vi "適應性控制_輸入權重係數+數位積分_隔振(實際控制).vi"() -> ()   [LabVIEW 2010]
uses:
  <vilib>/DAQmx/read.llb/DAQmx Read (Analog DBL 1Chan 1Samp).vi
  <vilib>/DAQmx/write.llb/DAQmx Write (Analog DBL 1Chan 1Samp).vi
  <vilib>/DAQmx/create/channels.llb/DAQmx Create Channel (AI-Voltage-Basic).vi
  <vilib>/DAQmx/configure/timing.llb/DAQmx Timing (Sample Clock).vi
  <vilib>/DAQmx/create/channels.llb/DAQmx Create Channel (AO-Voltage-Basic).vi
  <vilib>/daqmx/miscellaneous.llb/DAQmx Fill In Error Info.vi
  <vilib>/measure/maspectr.llb/FFT Spectrum (Mag-Phase) for 1 Chan.vi
  <vilib>/measure/NI_MAPro.lvlib
panel:
  in  "averaging parameters":T1={"averaging mode"=enum."No averaging", "weighting mode"=enum."Exponential", "number of averages"=10} {"number of averages" min=1}
  in  "I增益":dbl
  out "magnitude":cluster{"f0":dbl, "df":dbl, "magnitude":dbl[]} {"magnitude" format="%.2p"; "f0" format="%0.2p"; "df" format="%0.2p"}
  out "x >= y?":bool
  out "Waveform Graph":cluster{"f0":dbl, "df":dbl, "magnitude":dbl[]}(graph)
  in  "DAQ input":tag
  in  "DAQ output":tag
  in  "平均數":i32=1
  in  "ÂoDC«á©ñ¤j":dbl=1.0
  in  "Kp":dbl
  out "當下誤差":dbl=0.1 format="%#_13g"
  out "模擬輸入x(t)":dbl[][](graph)
  out "理想與FIR輸出":dbl[][](graph)
  out "message":string=" INSTRUCTIONS:\r\rNormal Use:  When using subVIs that incorporate the error in/error out (or error I/O) structure, place this handler where you want to inform the user of an error, typically at the end of the I/O data path, as the last action of the program.  If the error in error? is ERROR, the handler creates a message describing the error and its source.  If the type of dialog = 1 (default), the message is displayed to the user, who can only acknowedge it.  If the type = 2, the user can acknowledge the message or abort execution; aborting a program with active I/O is not recommended.  If the type = 0, no message is displayed; this is used to process the error programmatically, and the error out cluster elements are wired to individual terminals for that reason.  \r\rOther Use:\n\r\nlocal testing.  To test the error code of a subVI or function that does not have the error I/O structure, you can wire its error code and a source string to the local error code and error source inputs.  If error in error? indicates no error and error code is not equal to 0, the local code and source are substituted for the error in values, and error? is set TRUE (ERROR)."
  out "誤差":dbl(graph)
  out "while平均運行時間":dbl
  out "收斂time":dbl
  out "各頻率誤差已達標準":bool
  in  "各頻率誤差低於多少亮燈":dbl=0.1 format="%#_13g"
  in  "order":i32=100
  in  "取樣頻率":dbl=100.0 min=1.0 max=1000.0 step=1.0
  in  "stop":bool
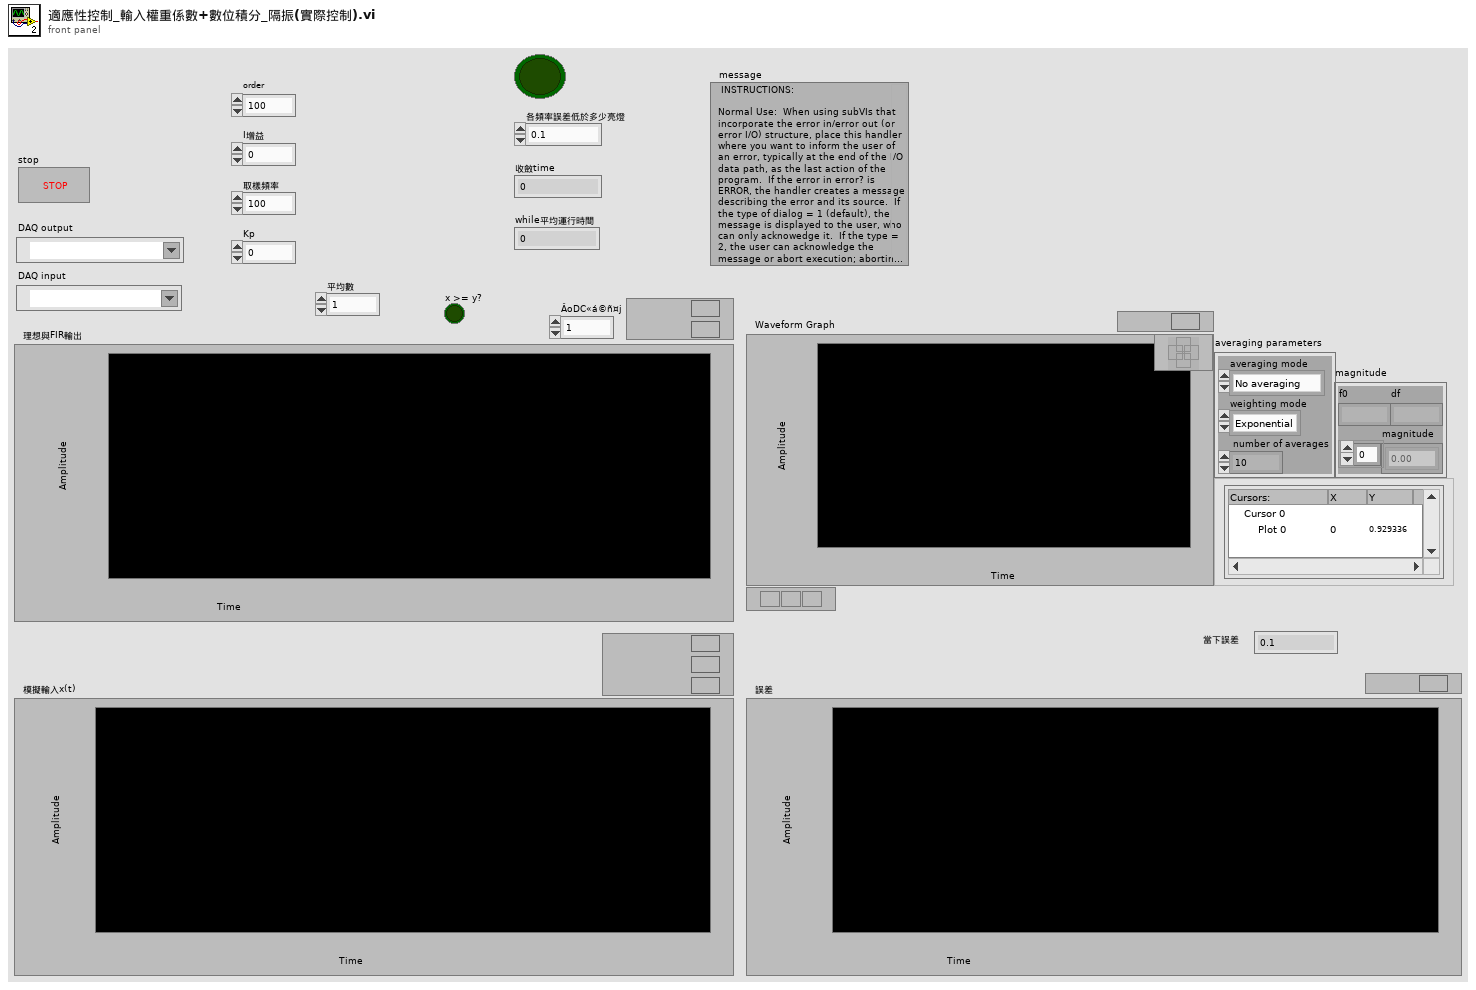
[diagram p1: front panel]
types:
  T1 = cluster{"averaging mode":enum16{"No averaging", "Vector averaging", "RMS averaging", "Peak hold"}, "weighting mode":enum16{"Linear", "Exponential"}, "number of averages":u32}
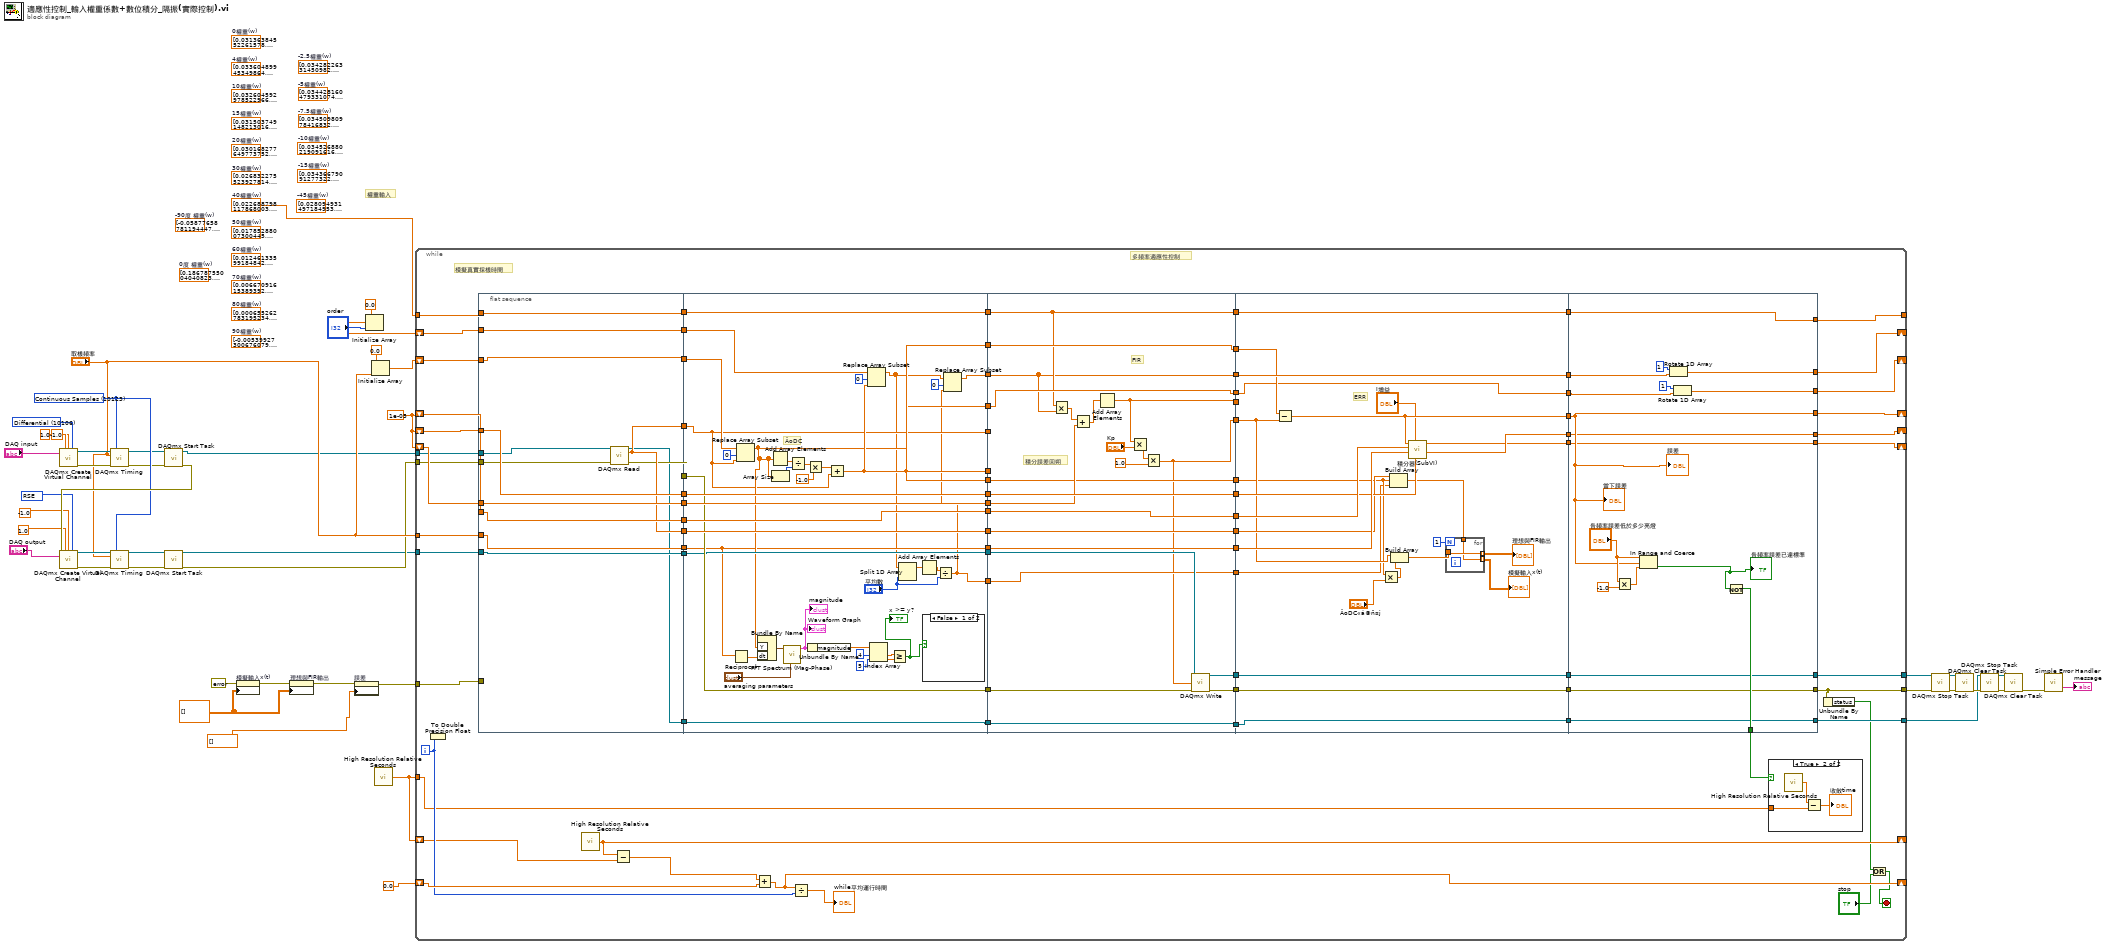
[diagram p0: block diagram]
diagram:
  (unwired) dbl[] [0.028094931497184953, 0.027318051498735518, 0.02651879137319172, 0.02569807185586792, 0.024856829443012252, 0.023996015437237974, 0.023116594986324603, 0.022219546115147443, 0.021305858750507205, 0.020376533738653148, 0.019432581855336542, 0.01847502280827197, 0.01750488423195552, 0.01652320067484008, 0.015531012578964592, 0.014529365252202192, 0.013519307833396409, 0.012501892250745314, 0.011478172173896465, 0.010449201960325366, 0.009416035596672211, 0.00837972563582886, 0.007341322130674419, 0.0063018715654710395, 0.005262415786041815, 0.004223990929959873, 0.003187626358084177, 0.002154343588880318, 0.0011251552370595153, 0.00010106395816484767, -0.0009169385991820944, -0.001927872831580498, -0.002930772207829844, -0.00392468428265997, -0.004908671695227361, -0.00588181315034755, -0.006843204380400101, -0.007791959085817819, -0.008727209852058984, -0.009648109040964999, -0.010553829654414855, -0.011443566168217257, -0.012316535334218085, -0.013171976948660059, -0.014009154584890944, -0.014827356288608607, -0.015625895233920068, -0.016404110338605567, -0.017161366837102645, -0.017897056809864115, -0.018610599667884493, -0.019301442591371253, -0.019969060921687886, -0.020612958505892797, -0.021232667993384594, -0.02182775108436404, -0.022397798730027247, -0.02294243128460723, -0.02346129860960119, -0.023954080130721905, -0.024420484848320073, -0.02486025130223469, -0.025273147492222828, -0.025658970755303042, -0.026017547601540937, -0.026348733509958266, -0.026652412686409777, -0.02692849778540182, -0.02717692959795794, -0.02739767670772351, -0.027590735117597045, -0.027756127849228453, -0.027893904517764606, -0.02800414088424619, -0.028086938388049064, -0.028142423661741165, -0.028170748030678785, -0.02817208699960081, -0.028146639728389652, -0.02809462849906762]  # -45權重(w)
  (unwired) dbl[] [-0.00539927300676079, -0.004574244171263112, -0.0037509801609765317, -0.0029302816336518054, -0.002112938043582804, -0.0012997269243527085, -0.0004914132117880658, 0.00031125139289816275, 0.001107529020049304, 0.00189669618911319, 0.0026780443275469003, 0.003450880252045411, 0.004214526613258243, 0.004968322305336847, 0.005711622841811576, 0.006443800699430544, 0.007164245631703628, 0.00787236495397947, 0.008567583801947519, 0.009249345365491084, 0.00991711109983541, 0.01057036091592068, 0.01120859335190286, 0.011831325727629191, 0.01243809428386606, 0.013028454307965948, 0.013601980247555422, 0.014158265813706777, 0.014696924074924332, 0.015217587543133453, 0.015719908252715378, 0.01620355783346848, 0.016668227578224903, 0.017113628505685517, 0.01753949141887445, 0.01794556695946006, 0.01833162565802534, 0.018697457980225856, 0.019042874368621635, 0.01936770527983496, 0.019671801216557375, 0.019955032753801623, 0.02021729055869038, 0.02045848540297177, 0.020678548167360374, 0.02087742983672937, 0.021055101485111045, 0.02121155424941127, 0.021346799290705574, 0.02146086774194928, 0.02155381064092829, 0.02162569884726334, 0.021676622942297136, 0.02170669311070986, 0.02171603900274138, 0.02170480957594453, 0.021673172915446008, 0.021621316031757785, 0.02154944463526281, 0.0214577828865742, 0.021346573122078515, 0.021216075554065406, 0.02106656794496731, 0.02089834525535277, 0.0207117192654478, 0.020507018170093982, 0.02028458614719378, 0.020044782899845154, 0.019787983172514116, 0.019514576241749453, 0.019224965382103488, 0.01891956730807669, 0.018598811593062675, 0.01826314006642601, 0.017913006189998734, 0.017548874415424298, 0.017171219523929186, 0.01678052595022868, 0.016377287092401892, 0.015962004609691362]  # 90權重(w)
  (unwired) dbl[] [0.000655262783195234, 0.0014201078745085935, 0.0021774020972579466, 0.002926443888983223, 0.0036665482827068136, 0.004397047528653455, 0.005117291670540145, 0.005826649076006129, 0.006524506921026103, 0.0072102716284213626, 0.007883369260847498, 0.008543245868894885, 0.009189367795184315, 0.009821221935571046, 0.010438315958788755, 0.011040178486057891, 0.011626359232366039, 0.012196429111279456, 0.012749980305275018, 0.01328662630369608, 0.013806001910512301, 0.014307763224125022, 0.014791587591492175, 0.01525717353885328, 0.015704240681322403, 0.016132529613576106, 0.016541801783804003, 0.01693183935301074, 0.017302445041656855, 0.017653441965513737, 0.017984673462477143, 0.018296002911941722, 0.01858731354818533, 0.018858508269058803, 0.019109509441096958, 0.01934025870201465, 0.01955071676136483, 0.019740863199973476, 0.019910696268596727, 0.020060232686074937, 0.020189507437109056, 0.020298573569623023, 0.02038750199153626, 0.02045638126663941, 0.020505317409132445, 0.020534433676282337, 0.020543870358546826, 0.02053378456642888, 0.020504350013242287, 0.020455756792913834, 0.02038821115188715, 0.02030193525416185, 0.0201971669384727, 0.02007415946660244, 0.019933181261818818, 0.01977451563643863, 0.01959846050754766, 0.019405328099933034, 0.019195444635336765, 0.018969150007184216, 0.018726797440022064, 0.018468753132954787, 0.018195395886468565, 0.01790711671211353, 0.017604318424615885, 0.017287415216095867, 0.016956832212185698, 0.016613005009947363, 0.016256379197624637, 0.015887409856384125, 0.015506561044327013, 0.015114305263196064, 0.014711122908324714, 0.014297501702517113, 0.013873936114681207, 0.01344092676416721, 0.012998979811898303, 0.01254860633950505, 0.012090321717796058, 0.011624644966018761]  # 80權重(w)
  (unwired) dbl[] [0.00667091615389392, 0.0073531796215807205, 0.008022353499817968, 0.008677855658426154, 0.0093191252965615, 0.009945623446932242, 0.01055683343253673, 0.011152261275102226, 0.01173143605465801, 0.012293910219937266, 0.012839259849567968, 0.0133670848642776, 0.013877009190596819, 0.014368680876806187, 0.014841772162116167, 0.015295979500309196, 0.015731023539294408, 0.01614664905823473, 0.01654262486409535, 0.016918743649629534, 0.017274821814967204, 0.01761069925509673, 0.017926239115628573, 0.018221327519306194, 0.018495873265781063, 0.018749807507191584, 0.018983083402092395, 0.019195675750248362, 0.019387580610770918, 0.01955881490600148, 0.019709416013460674, 0.019839441348070867, 0.01994896793674781, 0.02003809198730413, 0.020106928453470334, 0.02015561059767175, 0.020184289553033544, 0.020193133885911513, 0.02018232916007052, 0.020152077503450435, 0.020102597178287, 0.02003412215517216, 0.019946901691477305, 0.019841199914387982, 0.019717295408651407, 0.019575480808984056, 0.0194160623969507, 0.019239359702002117, 0.019045705106238656, 0.01883544345237183, 0.018608931654259798, 0.018366538309320644, 0.01810864331206435, 0.017835637467933978, 0.017547922106607765, 0.0172459086938986, 0.016930018441365446, 0.016600681912763208, 0.0162583386264637, 0.015903436653009115, 0.015536432206992573, 0.01515778923250659, 0.014767978981454962, 0.014367479584085715, 0.013956775611178068, 0.013536357627390475, 0.013106721735366355, 0.012668369110286092, 0.012221805524647291, 0.011767540863162248, 0.011306088627763677, 0.010837965432821188, 0.01036369049078064, 0.009883785088553226, 0.009398772055093806, 0.008909175220725613, 0.00841551886887598, 0.007918327181006855, 0.007418123675629097, 0.006915430642395791]  # 70權重(w)
  (unwired) dbl[] [0.01246133599184842, 0.013041219831202504, 0.013602894406144423, 0.014145913686861338, 0.014669856948559828, 0.015174329133535792, 0.015658961166438435, 0.01612341022168393, 0.01656735994218592, 0.016990520608790343, 0.017392629260042803, 0.017773449762143567, 0.018132772829205633, 0.01847041599416169, 0.01878622353092701, 0.019080066328656997, 0.019351841719184283, 0.01960147325894746, 0.019828910466937345, 0.020034128520405686, 0.02021712791025534, 0.02037793405822041, 0.020516596898084622, 0.020633190423331605, 0.020727812203723175, 0.020800582873394126, 0.020851645593115937, 0.020881165489419887, 0.02088932907328999, 0.020876343641121745, 0.02084243666062208, 0.020787855144258918, 0.020712865012808217, 0.02061775045144026, 0.020502813260682387, 0.020368372204463133, 0.020214762357301148, 0.02004233445254702, 0.01985145423342024, 0.019642501808414096, 0.019415871012459316, 0.019171968775060666, 0.018911214496432904, 0.018634039432489067, 0.01834088608934769, 0.01803220762786084, 0.017708467278491697, 0.01737013776671445, 0.017017700748963114, 0.01665164625901359, 0.016272472164555577, 0.015880683633604304, 0.015476792610288682, 0.015061317299474863, 0.014634781659602443, 0.014197714903051736, 0.01375065100331456, 0.013294128208201897, 0.012828688558305545, 0.012354877409919147, 0.011873242961626859, 0.011384335783784626, 0.010888708350142303, 0.010386914570892993, 0.009879509326477619, 0.00936704800152902, 0.008850086018401487, 0.008329178369796334, 0.007804879150074156, 0.007277741084921289, 0.006748315059123063, 0.006217149642286703, 0.005684790612449048, 0.005151780477596648, 0.004618657995224534, 0.004085957690156384, 0.003554209370946196, 0.003023937645278717, 0.0024956614348826222, 0.0019698934905635845]  # 60權重(w)
  (unwired) dbl[] [0.01785288007300445, 0.018313549484099297, 0.01875146243947006, 0.019166321764041604, 0.01955785875766229, 0.019925833390966242, 0.020270034456919973, 0.02059027967701616, 0.02088641576122781, 0.021158318421011374, 0.021405892334826912, 0.021629071065836773, 0.021827816931648425, 0.02200212082617336, 0.02215200199389503, 0.0222775077570517, 0.022378713196462365, 0.022455720786945993, 0.022508659988498554, 0.02253768679459808, 0.022542983239220365, 0.022524756864332075, 0.022483240149813264, 0.02241868990792409, 0.022331386644584658, 0.022221633889865745, 0.022089757500200716, 0.021936104934927047, 0.021761044509828513, 0.021564964630406868, 0.021348273007631896, 0.021111395858927785, 0.020854777097133657, 0.020578877510134784, 0.02028417393380734, 0.019971158420829367, 0.01964033740782395, 0.01929223088316994, 0.018927371557704305, 0.01854630404037417, 0.018149584020758995, 0.017737777460210984, 0.017311459793187052, 0.016871215140176334, 0.016417635533441485, 0.015951320156614594, 0.01547287459900939, 0.014982910125334536, 0.014482042961323908, 0.013970893595633676, 0.013450086098201664, 0.012920247455119799, 0.012382006919929456, 0.011835995381132669, 0.011282844745594366, 0.010723187337414892, 0.010157655311766505, 0.00958688008311379, 0.009011491767180241, 0.008432118635978309, 0.007849386585186942, 0.007263918613140568, 0.006676334310689538, 0.006087249361190102, 0.0054972750499046215, 0.004907017782112015, 0.004317078609266263, 0.003728052762584605, 0.0031405291934967785, 0.0025550901204460315, 0.0019723105815968736, 0.0013927579930736271, 0.0008169917124283485, 0.0002455626071138371, -0.00032098737218195605, -0.0008821256134018418, -0.0014373292601635595, -0.0019860856238763302, -0.0025278925907399885, -0.0030622590233541505]  # 50權重(w)
  w1 = dbl[] [0.022688798117868003, 0.023016703123977605, 0.023318008487520508, 0.02359257453440416, 0.023840292415774466, 0.024061084118485853, 0.024254902434520387, 0.024421730888538103, 0.024561583622842255, 0.02467450523916157, 0.02476057059678428, 0.024819884566718728, 0.024852581741703586, 0.02485882610205748, 0.02483881063751958, 0.0247927569254129, 0.024720914665639287, 0.024623561173202368, 0.024501000829138836, 0.024353564490923844, 0.024181608863604643, 0.023985515833094145, 0.02376569176323148, 0.02352256675838937, 0.023256593893559507, 0.02296824841400089, 0.022658026906665633, 0.02232644644574225, 0.02197404371475412, 0.021601374107744833, 0.021209010812141927, 0.02079754387595296, 0.020367579261963257, 0.019919737891628254, 0.019454654681336437, 0.018972977573689306, 0.01847536656640235, 0.017962492741357045, 0.017435037296253165, 0.016893690581209736, 0.016339151142542342, 0.015772124775823664, 0.015193323590181596, 0.014603465085647513, 0.014003271245200621, 0.013393467642993524, 0.012774782570070415, 0.012147946178719771, 0.011513689646429045, 0.010872744360239406, 0.01022584112213084, 0.009573709375904217, 0.008917076455873666, 0.008256666857533158, 0.007593201530222381, 0.006927397191690429, 0.006259965664337748, 0.005591613232811757, 0.004923040022538848, 0.004254939398695444, 0.0035879973850543225, 0.002922892102086354, 0.0022602932236582547, 0.0016008614516365126, 0.0009452480076909429, 0.0002940941415857486, -0.00035196934474902294, -0.0009923225580571462, -0.0016263569601737743, -0.0022534758006542686, -0.002873094536206727, -0.0034846412374721723, -0.004087556983643082, -0.0046812962453512755, -0.0052653272561928215, -0.005839132373191945, -0.006402208426435722, -0.006954067058039844, -0.0074942350505364345, -0.008022254644699871]  # 40權重(w)
  (unwired) dbl[] [0.026832275523927814, 0.027017456806583375, 0.027173006485582622, 0.02729894675169174, 0.027395332150102945, 0.02746224939541744, 0.027499817148737792, 0.0275081857564142, 0.02748753695005452, 0.02743808350749108, 0.027360068874483043, 0.027253766747031807, 0.027119480614293475, 0.026957543262189007, 0.026768316237928816, 0.026552189275804685, 0.026309579684734425, 0.02604093169818175, 0.025746715787220296, 0.025427427937661357, 0.025083588892304436, 0.02471574335952802, 0.024324459189574908, 0.023910326520042404, 0.023473956892216173, 0.023015982340030425, 0.022537054453558754, 0.022037843419059178, 0.021519037037708133, 0.020981339725249404, 0.02042547149487626, 0.019852166925722864, 0.019262174119413035, 0.01865625364713688, 0.01803517748976458, 0.017399727973502165, 0.01675069670359472, 0.016088883498547667, 0.01541509532729882, 0.014730145251716288, 0.014034851376716938, 0.01333003581021883, 0.012616523635032894, 0.01189514189468816, 0.011166718595055088, 0.010432081723500766, 0.009692058287162894, 0.008947473371779927, 0.008199149222362706, 0.0074479043468326485, 0.006694552643594076, 0.005939902553851216, 0.0051847562393217165, 0.004429908785848688, 0.0036761474332641913, 0.002924250831717536, 0.0021749883245472954, 0.0014291192576526444, 0.0006873923152044775, -4.945511856778414e-05, -0.0007806975718707744, -0.0015056220725621578, -0.0022235287105953658, -0.0029337311762616222, -0.00363555727484346, -0.0043283494183292415, -0.005011465094861392, -0.005684277316604827, -0.0063461750467239, -0.006996563606149848, -0.0076348650608044615, -0.008260518589921348, -0.008872980836075177, -0.009471726237490099, -0.010056247343156193, -0.010626055111231917, -0.011180679191159846, -0.01171966818986646, -0.012242589922357074, -0.01274903164695937]  # 30權重(w)
  (unwired) dbl[] [0.030168277649773752, 0.0302046668904262, 0.030209285636136392, 0.030182317860428007, 0.030123980591716712, 0.03003452353476148, 0.0299142286568077, 0.029763409738362875, 0.029582411888611996, 0.029371611025521577, 0.029131413320757457, 0.028862254609605443, 0.028564599766165648, 0.028238942044167253, 0.02788580238384603, 0.027505728685415787, 0.02709929504976696, 0.02666710098711982, 0.026209770594477558, 0.025727951702820544, 0.025222314995103794, 0.024693553096219126, 0.02414237963620683, 0.023569528288104113, 0.022975751781926314, 0.02236182089638452, 0.02172852343004444, 0.02107666315372389, 0.020407058746018142, 0.019720542713925936, 0.019017960300617698, 0.01830016838245857, 0.01756803435744805, 0.01682243502728163, 0.016064255475275378, 0.01529438794240603, 0.014513730703735662, 0.013723186947471855, 0.012923663658902922, 0.012116070511410821, 0.011301318766718397, 0.010480320186468607, 0.009653985957161364, 0.008823225630392525, 0.007988946080242922, 0.007152050479562386, 0.006313437296782354, 0.005473999314766556, 0.004634622673086221, 0.0037961859349694128, 0.0029595591800416284, 0.002125603123833017, 0.001295168264889402, 0.00046909406018398695, -0.00035179187061121, -0.0011666745115700083, -0.001974752187379217, -0.0027752372704600383, -0.0035673568582946106, -0.004350353421019048, -0.005123485419448939, -0.005886027893795931, -0.006637273023420805, -0.007376530658040955, -0.008103128820877587, -0.0088164141842808, -0.009515752518415244, -0.01020052911362381, -0.010870149177111044, -0.011524038204601657, -0.012161642327635575, -0.012782428637159105, -0.013385885484060365, -0.013971522757276322, -0.014538872140078664, -0.015087487345112447, -0.015616944328725521, -0.016126841485087615, -0.016616799820557703, -0.017086463108704444]  # 20權重(w)
  (unwired) dbl[] [0.031503749148213016, 0.03146476198752651, 0.03139328837071151, 0.031289591702925085, 0.031153968477006574, 0.030986747802974807, 0.03078829090327016, 0.03055899057387441, 0.030299270611494605, 0.030009585207043703, 0.029690418305714755, 0.02934228293400063, 0.028965720494088843, 0.028561300026127726, 0.028129617438940747, 0.0276712947098461, 0.027186979054326554, 0.02667734206637921, 0.02614307883047204, 0.02558490700611989, 0.025003565886194703, 0.02439981543017418, 0.0237744352736317, 0.023128223715362408, 0.02246199668363435, 0.021776586683142047, 0.021072841724324977, 0.02035162423679804, 0.019613809968714403, 0.018860286873951155, 0.018091953989073248, 0.017309720302083907, 0.01651450361501605, 0.015707229402454878, 0.014888829668113798, 0.01406024180159235, 0.013222407437458793, 0.012376271318788368, 0.011522780167272895, 0.01066288156198606, 0.009797522828849044, 0.008927649942787526, 0.008054206444510454, 0.007178132373761786, 0.006300363220819022, 0.005421828897913179, 0.004543452732148049, 0.0036661504813840784, 0.002790829374439085, 0.0019183871768360052, 0.0010497112832038979, 0.00018567783730916583, -0.0006728491194340122, -0.0015250184702561224, -0.0023699928155388236, -0.0032069492350738082, -0.004035080019736721, -0.004853593372358783, -0.005661714077693553, -0.00645868414148456, -0.007243763398742078, -0.008016230091429651, -0.008775381415848047, -0.009520534040080632, -0.010251024591931801, -0.010966210117847996, -0.011665468513360635, -0.012348198925629592, -0.013013822128695033, -0.013661780872068232, -0.014291540203302477, -0.014902587765190977, -0.015494434068234024, -0.01606661273900806, -0.016618680745049255, -0.017150218596845006, -0.017660830527494082, -0.01815014465056855, -0.018617813096664708, -0.019063512129106033]  # 15權重(w)
  (unwired) dbl[] [0.032604592978522966, 0.032490299881371074, 0.03234304676422258, 0.03216317471496727, 0.03195105772468281, 0.03170710213045929, 0.03143174602491757, 0.0311254586327216, 0.030788739654430193, 0.030422118578084203, 0.030026153958981606, 0.0296014326681496, 0.029148569110089884, 0.02866820441043807, 0.028161005574252856, 0.027627664615721196, 0.027068897660143074, 0.026485444019145113, 0.02587806524014163, 0.025247544131156416, 0.024594683762192773, 0.023920306444426286, 0.02322525268857691, 0.022510380143895635, 0.021776562519282866, 0.021024688488128676, 0.020255660578540044, 0.019470394050686273, 0.018669815763057967, 0.017854863029491415, 0.017026482468862052, 0.016185628849388744, 0.015333263929539646, 0.014470355297536515, 0.013597875211493205, 0.012716799442220218, 0.011828106120730002, 0.010932774592466754, 0.010031784280263027, 0.009126113557995103, 0.008216738636864635, 0.007304632466186566, 0.006390763650498811, 0.005476095384740476, 0.004561584409165472, 0.0036481799855704734, 0.0027368228963221084, 0.001828444467565326, 0.0009239656178886064, 2.4295933608189456e-05, -0.0008696672282818424, -0.0017570396085662334, -0.0026369508848650886, -0.0035085454806047943, -0.004370983343338324, -0.005223440691969621, -0.006065110732552799, -0.006895204342450429, -0.007712950722743131, -0.008517598018886364, -0.009308413909706393, -0.01008468616491852, -0.010845723171431572, -0.011590854428780124, -0.01231943101408886, -0.013030826017033714, -0.013724434945314352, -0.014399676101189576, -0.015055990929663005, -0.015692844338928588, -0.016309724993698246, -0.01690614558204773, -0.017481643056407904, -0.018035778849332374, -0.018568139064650897, -0.019078334644602582, -0.01956600151352087, -0.020030800698613984, -0.02047241842834564, -0.020890566208901486]  # 10權重(w)
  (unwired) dbl[] [0.03360489945349864, 0.033401122697626545, 0.0331641419081741, 0.032894388258261034, 0.03259232530867979, 0.032258448355600065, 0.031893283746068264, 0.03149738816175537, 0.031071347871449037, 0.030615777952848307, 0.03013132148426028, 0.029618648706870785, 0.02907845615831185, 0.02851146577832233, 0.027918423987361343, 0.02730010073910487, 0.026657288547829956, 0.025990801491763648, 0.025301474193544157, 0.02459016077902413, 0.023857733815712896, 0.02310508323223205, 0.02233311522022953, 0.02154275112026902, 0.020734926293274614, 0.019910588979183054, 0.0190706991445037, 0.018216227320552142, 0.01734815343416897, 0.01646746563277857, 0.015575159105681285, 0.014672234903501667, 0.013759698757740281, 0.01283855990238848, 0.011909829899573407, 0.010974521471198293, 0.010033647338529341, 0.009088219071663123, 0.008139245950775385, 0.007187733841015768, 0.006234684082861911, 0.0052810923996928555, 0.004327947824273103, 0.0033762316457669342, 0.0024269163788202667, 0.0014809647561603134, 0.0005393287460672937, -0.0003970514040266215, -0.0013272480966614044, -0.0022503472851550773, -0.003165449345162201, -0.004071669916169326, -0.004968140712226453, -0.005854010301329044, -0.006728444852977508, -0.007590628853555011, -0.008439765789272198, -0.00927507879653338, -0.010095811279679394, -0.010901227496158857, -0.011690613109268376, -0.01246327570868491, -0.013218545299091325, -0.01395577475726373, -0.014674340258048237, -0.015373641669712489, -0.01605310291919537, -0.016712172327822527, -0.017350322918074423, -0.017967052692027217, -0.01856188488208504, -0.019134368174642136, -0.019684076907303134, -0.02021061124028655, -0.0207135973026234, -0.021192687313744206, -0.021647559681027287, -0.022077919073848692, -0.022483496474651924, -0.022864049207520207]  # 4權重(w)
  (unwired) dbl[] [0.03436679091277322, 0.033896935329659955, 0.03339544330543104, 0.03286299772349098, 0.0323003100148073, 0.03170811928611475, 0.031087191420834, 0.030438318153265108, 0.029762316116657195, 0.02906002586582564, 0.02833231087505625, 0.02758005651209314, 0.026804168989089033, 0.026005574291463284, 0.025185217085698357, 0.024344059607170808, 0.023483080529205114, 0.022603273814611514, 0.021705647551049728, 0.02079122277164197, 0.019861032262336945, 0.018916119357597426, 0.017957536726070342, 0.01698634514795136, 0.016003612285839505, 0.015010411450928497, 0.014007820366441468, 0.012996919930266412, 0.011978792978792577, 0.01095452305398442, 0.009925193175756849, 0.008891884621736412, 0.007855675716500315, 0.006817640632388642, 0.005778848203971962, 0.004740360758238829, 0.0037032329625338533, 0.0026685106922374616, 0.001637229920123448, 0.0006104156292681232, -0.0004109192486902176, -0.0014257748682273066, -0.0024331654759244467, -0.003432120386259613, -0.004421684925793986, -0.005400921344470465, -0.0063689096928667074, -0.00732474866437905, -0.008267556401449527, -0.009196471265091039, -0.010110652567106861, -0.011009281264546734, -0.011891560616084788, -0.012756716800146414, -0.013603999494752177, -0.014432682419179301, -0.015242063837674966, -0.01603146702557367, -0.016800240698290718, -0.017547759403768872, -0.018273423879051242, -0.018976661371743014, -0.019656925927198386, -0.02031369864233602, -0.020946487887036187, -0.02155482949412064, -0.02213828691893767, -0.02269645136960095, -0.023228941908932196, -0.023735405529160012, -0.02421551720040211, -0.024668979893954494, -0.025095524581353734, -0.025494910210163126, -0.025866923657366266, -0.026211379661216682, -0.0265281207323179, -0.026817017044660798, -0.027077966307271887, -0.02731089361706443]  # -15權重(w)
  (unwired) dbl[] [0.034526880219091616, 0.03412341864898172, 0.03368756605967875, 0.033219945097828364, 0.0327212083001866, 0.032192037266465495, 0.03163314180320718, 0.031045259039270627, 0.030429152513570715, 0.029785611235773373, 0.029115448720699766, 0.028419501997273684, 0.027698630592902118, 0.026953715494255452, 0.026185658085486535, 0.0253953790649998, 0.02458381734196095, 0.023751928913807844, 0.022900685726105974, 0.022031074516161844, 0.021144095641884235, 0.020240761897454832, 0.019322097317439477, 0.018389135971036214, 0.017442920748222086, 0.016484502139613912, 0.015514937011914403, 0.014535287380858975, 0.013546619183621182, 0.01255000105266479, 0.011546503093056213, 0.010537195665268716, 0.009523148175516343, 0.008505427875653192, 0.007485098674665999, 0.006463219963761539, 0.005440845457025946, 0.004419022049586188, 0.0033987886951570485, 0.0023811753047935256, 0.0013672016685999822, 0.00035787640206595575, -0.0006458040813892314, -0.0016428565701778488, -0.0026323120252304062, -0.0036132165203381205, -0.004584632150998247, -0.005545637910732174, -0.0064953305339711795, -0.007432825304733386, -0.00835725683044721, -0.009267779780405385, -0.010163569588465841, -0.011043823119743106, -0.011907759301159792, -0.012754619715850131, -0.013583669161522685, -0.01439419617300103, -0.015185513509264685, -0.015956958605408186, -0.01670789399002304, -0.01743770766858901, -0.018145813473524917, -0.018831651381614266, -0.0194946877995657, -0.020134415818512167, -0.020750355438276826, -0.021342053762257614, -0.021909085163793102, -0.022451051424867582, -0.022967581848012272, -0.02345833334224216, -0.023922990483841503, -0.024361265552788877, -0.024772898545570136, -0.02515765716509303, -0.025515336788370674, -0.025845760412594055, -0.026148778580164896, -0.026424269283206715]  # -10權重(w)
  (unwired) dbl[] [0.03450980978416832, 0.03414068213407085, 0.03373887697229963, 0.033304985060518856, 0.032839627632241304, 0.032343455591603294, 0.03181714868245221, 0.031261414628338945, 0.030676988244049748, 0.030064630519381044, 0.02942512767590848, 0.02875929019757547, 0.028067951835988245, 0.02735196859137534, 0.026612217670238934, 0.02584959642080119, 0.02506502124741905, 0.024259426505217525, 0.02343376337626524, 0.022588998728690645, 0.021726113960207002, 0.020846103827589172, 0.019949975263709882, 0.019038746183808974, 0.01811344428273319, 0.017175105824936445, 0.016224774429084345, 0.015263499849153647, 0.014292336753955824, 0.013312343507043382, 0.01232458094898808, 0.011330111184031958, 0.010329996373123205, 0.00932529753534598, 0.00831707335974466, 0.007306379029525169, 0.00629426506058004, 0.005281776156255329, 0.004269950080219724, 0.003259816549243291, 0.0022523961476243696, 0.0012486992649274908, 0.00024972505860979, -0.0007435395569781286, -0.0017301208938313543, -0.0027090594444901584, -0.003679410806032004, -0.004640246572804748, -0.00559065519696992, -0.006529742816048176, -0.007456634046782828, -0.008370472744764462, -0.009270422729380862, -0.010155668473784258, -0.011025415759683297, -0.011878892296887667, -0.012715348307643613, -0.01353405707590471, -0.01433431546178325, -0.0151154443815203, -0.015876789253396428, -0.016617720410082665, -0.017337633478001786, -0.018035949724321095, -0.01871211637225937, -0.019365606885418447, -0.01999592122189097, -0.020602586058912808, -0.02118515498884159, -0.02174320868725039, -0.022276355053919873, -0.022784229327501525, -0.023266494174608042, -0.023722839754063384, -0.024152983757012157, -0.024556671423558878, -0.02493367553656561, -0.02528379639319836, -0.025606861754765523, -0.025902726775350212]  # -7.5權重(w)
  (unwired) dbl[] [0.034428160479331074, 0.03409402943460197, 0.0337269955307479, 0.03332761655701684, 0.03289648129673356, 0.0324342087543726, 0.03194144735230872, 0.03141887409782341, 0.03086719372099331, 0.030287137784143693, 0.029679463763615053, 0.02904495410464373, 0.02838441525023091, 0.02769867664493668, 0.026988589714608782, 0.026255026823126488, 0.025498880207308658, 0.02472106089121793, 0.02392249758115134, 0.023104135542695803, 0.022266935461288377, 0.021411872287793884, 0.02053993407068117, 0.01965212077644314, 0.018749443099965565, 0.01783292126660725, 0.0169035838278067, 0.0159624664520739, 0.015010610713267576, 0.01404906287809304, 0.01307887269477501, 0.012101092184886796, 0.011116774440319195, 0.010126972427378016, 0.0091327377999887, 0.008135119723970605, 0.007135163714317525, 0.006133910487383202, 0.0051323948298275975, 0.004131644486123594, 0.0031326790663613485, 0.002136508976015656, 0.0011441343692599993, 0.00015654412732504767, -0.000825285136696868, -0.0018003900453006309, -0.0027678213950766122, -0.0037266450651958216, -0.004675942894904573, -0.005614813529179359, -0.006542373231811927, -0.0074577566653156934, -0.008360117637163348, -0.009248629811986972, -0.010122487389483674, -0.010980905747890011, -0.011823122052988681, -0.012648395832723345, -0.013456009517587806, -0.01424526894705347, -0.015015503842378071, -0.015766068246217606, -0.016496340929531575, -0.01720572576633056, -0.01789365207686505, -0.018559574939901097, -0.019202975474754608, -0.019823361093791545, -0.020420265726105148, -0.02099325001310105, -0.021541901476717334, -0.022065834660997503, -0.022564691247728516, -0.02303814014683174, -0.023485877562170153, -0.02390762703341159, -0.02430313945454922, -0.024672193069648542, -0.025014593446346323, -0.025330173427595998]  # -5權重(w)
  (unwired) dbl[] [0.03428226331450982, 0.03398371886005176, 0.03365210760572737, 0.033287953351065006, 0.03289181135276715, 0.0324642675824135, 0.03200593795326185, 0.03151746751670628, 0.030999529628997463, 0.030452825088884118, 0.02987808124689916, 0.02927605108706395, 0.028647512281859522, 0.02799326622137002, 0.027314137017582025, 0.026610970484884425, 0.025884633097891106, 0.02513601092778113, 0.024366008558418903, 0.023575547983594614, 0.022765567486792704, 0.021937020504968402, 0.021090874477877698, 0.020228109684573618, 0.01934971806874092, 0.018456702054598265, 0.01755007335515381, 0.01663085177464057, 0.015700064007006517, 0.01475874243236193, 0.013807923913321477, 0.01284864859319294, 0.011881958697979565, 0.010908897344165717, 0.009930507354251763, 0.008947830081988283, 0.007961904249238738, 0.006973764796366876, 0.005984441748002569, 0.004994959095991816, 0.004006333701276469, 0.0030195742163800616, 0.002035680030103744, 0.0010556402359496806, 8.043262570134233e-05, -0.0008889772905079723, -0.0018516372364083802, -0.002806609092965892, -0.0037529697919022674, -0.004689812178464137, -0.005616245842659207, -0.006531397918294134, -0.007434413849265338, -0.008324458122670214, -0.009200714968419836, -0.010062389025145153, -0.01090870597229605, -0.011738913128436095, -0.012552280015830844, -0.013348098891521405, -0.014125685245157046, -0.014884378263938939, -0.015623541265096633, -0.01634256209638034, -0.017040853505103835, -0.017717853476321228, -0.018373025540752208, -0.019005859053106727, -0.01961586944146861, -0.020202598428425114, -0.02076561422461871, -0.021304511695408753, -0.021818912501313393, -0.02230846521289356, -0.022772845400715492, -0.023211755701008682, -0.02362492585760606, -0.024012112740719495, -0.02437310034307015, -0.024707699753859873]  # -2.5權重(w)
  (unwired) dbl[] [0.03136384552261578, 0.03122796662859831, 0.03106127147498808, 0.03086392654110037, 0.030636128549990916, 0.030378104272370535, 0.030090110300876084, 0.029772432794913584, 0.029425387196335882, 0.029049317916230492, 0.02864459799313286, 0.02821162872300296, 0.027750839261329648, 0.027262686197763703, 0.02674765310369236, 0.026206250053211824, 0.025639013117966816, 0.025046503836359924, 0.024429308657656256, 0.023788038361531958, 0.023123327453643174, 0.02243583353781323, 0.021726236665456675, 0.020995238662889253, 0.020243562437182287, 0.01947195126125448, 0.018681168038903663, 0.017871994550507996, 0.017045230680140345, 0.01620169362486253, 0.015342217086977807, 0.014467650450043678, 0.01357885793945608, 0.012676717768437547, 0.011762121270270612, 0.010835972017636426, 0.009899184929926325, 0.008952685369411207, 0.007997408227158293, 0.007034296999601428, 0.006064302856674808, 0.005088383702431831, 0.004107503229076141, 0.003122629965339955, 0.0021347363201481497, 0.0011447976225137278, 0.00015379115861163982, -0.0008373047930174659, -0.0018275119271818313, -0.002815852877717708, -0.003801352182179886, -0.004783037244591619, -0.0057599392953033455, -0.006731094347013476, -0.007695544146007186, -0.008652337117675322, -0.009600529305379262, -0.010539185301737208, -0.011467379171411534, -0.012384195364487377, -0.013288729619542205, -0.014180089855514473, -0.01505739705149305, -0.015919786113558387, -0.016766406727821617, -0.017596424198820744, -0.018409020272446435, -0.019203393942586498, -0.01997876224069315, -0.020734361007498613, -0.02146944564611083, -0.02218329185575701, -0.022875196345442956, -0.023544477526829515, -0.02419047618564644, -0.024812556130974252, -0.02541010482176247, -0.025982533969962633, -0.026529280119684737, -0.027049805201806457]  # 0權重(w)
  (unwired) dbl[] [0.18678755004040823, 0.17882619748458314, 0.170712296455689, 0.16245257152505876, 0.15405454867553942, 0.14552523682324905, 0.13687159530574372, 0.12810196462388707, 0.11922362147035999, 0.11024393073088701, 0.10117036364485271, 0.09201149209306575, 0.08277436332911685, 0.07346739409850038, 0.06409841525561331, 0.05467582605915196, 0.04520705780003369, 0.03570079633951639, 0.02616517534237316, 0.016608099867348597, 0.007037550190427917, -0.002537488532805972, -0.012109386514070251, -0.021670078710663815, -0.031211136355664814, -0.04072404103843337, -0.050201506295751895, -0.059634697247062, -0.06901578876295462, -0.07833678686397391, -0.0875896165139027, -0.09676628530049372, -0.1058592127633476, -0.11486053312230449, -0.12376230508663352, -0.13255713450591536, -0.1412373426283469, -0.1497958727547784, -0.15822474190263155, -0.1665175154150831, -0.1746667650614144, -0.18266518234592094, -0.19050584543113128, -0.1981828435843626, -0.2056888768059049, -0.2130178209590218, -0.22016340348000582, -0.22711953829571419, -0.233880164162633, -0.24043951812605066, -0.2467920977101983, -0.25293205077048525, -0.2588545397521522, -0.2645544847915611, -0.27002654535583903, -0.2752661953902621, -0.28026944958627037, -0.28503187047512585, -0.28954881763286344, -0.29381678537090966, -0.29783232335913956, -0.30159129471393037, -0.3050912331475972, -0.30832924646728915, -0.3113020963534453, -0.3140069410480377, -0.31644199138653817, -0.3186047046785827, -0.3204935982376899, -0.32210684992236727, -0.32344335057664403, -0.3245013187862961, -0.3252801022894491, -0.32577926591498596, -0.32599826290987993, -0.32593663650954463, -0.32559487153422917, -0.3249726147434439, -0.3240708551869918, -0.3228901701852509]  # 0度 權重(w)
  (unwired) dbl[] [-0.05877658781194447, -0.05880165783072071, -0.058769626713902144, -0.05868052843544654, -0.05853445290663261, -0.05833154600716313, -0.05807200513047942, -0.05775609051408422, -0.05738411490100067, -0.05695643829566999, -0.05647347561480095, -0.05593570222205698, -0.05534364366063041, -0.0546978771243554, -0.05399903471184836, -0.05324779605889828, -0.052444887701321614, -0.05159109221709506, -0.050687246789522196, -0.04973422883689582, -0.04873296289280662, -0.04768442344356334, -0.046589627008202315, -0.04544963505892205, -0.044265561327572645, -0.043038556514139834, -0.041769807581880536, -0.04046054418500069, -0.03911204002747684, -0.03772560321594224, -0.0363025799259075, -0.03484435512137173, -0.033352340191170726, -0.03182797732145333, -0.030272749521124433, -0.02868816831319295, -0.027075769660101768, -0.025437116513894426, -0.02377379954828862, -0.022087426486926968, -0.020379633339138514, -0.018652081796517977, -0.01690644743242602, -0.01514441726000822, -0.013367701416755104, -0.01157802234878765, -0.009777114554821144, -0.007966727150988276, -0.006148619219587733, -0.00432454880331794, -0.0024962812704839394, -0.0006655945165545307, 0.0011657354252903728, 0.002995933356237631, 0.004823221823050019, 0.006645830331619849, 0.00846199503756085, 0.010269953129429738, 0.012067944536500928, 0.01385422736721719, 0.015627071128350007, 0.01738475403707428, 0.01912557209081219, 0.020847837381648134, 0.022549872651853698, 0.02423002464683928, 0.02588666747979125, 0.027518193376758496, 0.029123015099837102, 0.03069957472506095, 0.032246340970037195, 0.03376180823956406, 0.035244507411115795, 0.036693002110996215, 0.038105881963939006, 0.039481769906701984, 0.04081933200018057, 0.042117268135363845, 0.04337431575808651, 0.04458925443984995]  # -90度 權重(w)
  w29 = 10123 items=["Finite Samples"=10178, "Continuous Samples"=10123, "Hardware Timed Single Point"=12522] ("sample mode")
  w26 = 10083 items=["Default"=-1, "RSE"=10083, "Differential"=10106, "Pseudodifferential"=12529] ("output terminal configuration")
  w25 = 10106 items=["default"=-1, "RSE"=10083, "NRSE"=10078, "Differential"=10106, "Pseudodifferential"=12529] ("input terminal configuration")
  w37 = 1e-05 ("x")
  w33 = dbl[][] [] ("History Data")
  # "權重輸入"
  n1 = call-poly <vilib>:"DAQmx Create Virtual Channel.vi"("maximum value"=1.0, "minimum value"=-1.0, "input terminal configuration"=w25, "physical channels"="DAQ input") -> ("task out"=w17:refnum<k21>, "error out"=w20:errorcluster)  [unwired: 10 in]
  n2 = call-poly <vilib>:"DAQmx Timing.vi"("task/channels in"=w17, "sample mode"=w29, "rate"="取樣頻率", "error in"=w20) -> ("task out"=w18:refnum<k21>, "error out"=w19:errorcluster)  [unwired: 10 in]
  n3 = call <vilib>:"DAQmx Start Task.vi"("task/channels in"=w18, "error in"=w19) -> ("task out"=w15:refnum<k21>, "error out"=w32:errorcluster)  [unwired: 12 in]
  n4 = call-poly <vilib>:"DAQmx Create Virtual Channel.vi"("maximum value"=1.0, "minimum value"=-1.0, "output terminal configuration"=w26, "physical channels"="DAQ output", "error in"=w32) -> ("task out"=w24:refnum<k21>, "error out"=w21:errorcluster)  [unwired: 9 in]
  n5 = call-poly <vilib>:"DAQmx Timing.vi"("task/channels in"=w24, "sample mode"=w29, "rate"="取樣頻率", "error in"=w21) -> ("task out"=w23:refnum<k21>, "error out"=w22:errorcluster)  [unwired: 10 in]
  n6 = call <vilib>:"DAQmx Start Task.vi"("task/channels in"=w23, "error in"=w22) -> ("task out"=w13:refnum<k21>, "error out"=w14:errorcluster)  [unwired: 12 in]
  n7 = property on="模擬輸入x(t)" class="WFChart (strict)"(error in=errorcluster {"status"=FALSE, "code"=0, "source"=""} ("error constant"), "History Data"=w33) -> (error out=w41:errorcluster)  [unwired: 1 in, 1 out]
  n8 = property on="理想與FIR輸出" class="WFChart (strict)"(error in=w41, "History Data"=w33) -> (error out=w42:errorcluster)  [unwired: 1 in, 1 out]
  n9 = property on="誤差" class="WFChart (strict)"(error in=w42, "History Data"=dbl[] []) -> (error out=w44:errorcluster)  [unwired: 1 in, 1 out]
  n10 = Initialize Array(0.0 ("element"), "order") -> (w36:dbl[])
  n11 = Initialize Array(0.0 ("element"), "取樣頻率") -> (w34:dbl[])
  n12 = call <vilib>:"High Resolution Relative Seconds.vi"() -> ("relative seconds"=w46:dbl)
  n13 = while {
    shift-right: [w105] -> _
    shift-left: w36 -> [w130]
    tunnel: w46 -> [w113]
    shift-right: [w114] -> _
    shift-left: w46 -> [w112]
    shift-right: [w115] -> _
    shift-left: 0.0 -> [w117]
    tunnel: w44 -> [w109]
    shift-right: [w103] -> _
    shift-left: w37 -> [w99]
    shift-right: [w95] -> _
    shift-left: w37 -> [w90]
    shift-right: [w89] -> _
    shift-left: w37 -> [w85]
    tunnel: "取樣頻率" -> [w84]
    tunnel: w1 -> [w125]
    tunnel: [w79] -> _
    shift-right: [w76] -> _
    shift-left: w34 -> [w78]
    tunnel: w15 -> [w68]
    tunnel: w14 -> [w67]
    tunnel: w13 -> [w66]
    tunnel: [w61] -> w7
    tunnel: [w51] -> w6
    tunnel: [w54] -> w5
    i -> [w116]
    stop <- w53 stop-if-true
    # "模擬真實採樣時間"
    # "多頻率適應性控制"
    n14 = To Double Precision Float(number=w116) -> ()  [unwired: 1 out]
    n15 = flat-sequence {
      tunnel: [w147] -> w131
      tunnel: w130 -> [w147]
      tunnel: [w138] -> w129
      tunnel: [w146] -> w126
      tunnel: w125 -> [w146]
      tunnel: w109 -> [_]
      tunnel: [w138] -> w106
      tunnel: [w145] -> w100
      tunnel: w99 -> [w145]
      tunnel: [w144] -> w96
      tunnel: w84 -> [w144]
      tunnel: [w143] -> w91
      tunnel: w90 -> [w143]
      tunnel: [w142] -> w86
      tunnel: w85 -> [w142]
      tunnel: [w137] -> w83
      tunnel: w78 -> [w141]
      tunnel: [w141] -> w77
      tunnel: w68 -> [w140]
      tunnel: w67 -> [w139]
      tunnel: w66 -> [w136]
      tunnel: [w136] -> w64
      tunnel: [w135] -> w57
      tunnel: w131 -> [w184]
      tunnel: w129 -> [w152]
      tunnel: [w150] -> w128
      tunnel: [w185] -> w127
      tunnel: w126 -> [w185]
      tunnel: [w178] -> w110
      tunnel: [w183] -> w107
      tunnel: w106 -> [w183]
      tunnel: [w181] -> w101
      tunnel: w100 -> [w181]
      tunnel: [w155] -> w97
      tunnel: w96 -> [w155]
      tunnel: [w180] -> w92
      tunnel: w91 -> [w180]
      tunnel: [w179] -> w87
      tunnel: w86 -> [w179]
      tunnel: w83 -> [w178]
      tunnel: [w170] -> w81
      tunnel: w77 -> [w176]
      tunnel: [w157] -> w73
      tunnel: [w170] -> w72
      tunnel: [w170] -> w70
      tunnel: [w148] -> w69
      tunnel: [w166] -> w65
      tunnel: w64 -> [w166]
      tunnel: [w165] -> w58
      tunnel: w57 -> [w165]
      tunnel: [w152] -> w48
      tunnel: w128 -> [w188]
      tunnel: w127 -> [w190]
      tunnel: [w190] -> w124
      tunnel: [w189] -> w123
      tunnel: [w188] -> w122
      tunnel: w110 -> [w195]
      tunnel: [w187] -> w108
      tunnel: w107 -> [w187]
      tunnel: [w208] -> w102
      tunnel: w101 -> [w208]
      tunnel: [w207] -> w98
      tunnel: w97 -> [w207]
      tunnel: [w206] -> w93
      tunnel: w92 -> [w206]
      tunnel: w87 -> [w204]
      tunnel: [w200] -> w82
      tunnel: w81 -> [w200]
      tunnel: [w186] -> w80
      tunnel: [w198] -> w74
      tunnel: w73 -> [w198]
      tunnel: w72 -> [w199]
      tunnel: [w199] -> w71
      tunnel: w70 -> [_]
      tunnel: w69 -> [w191]
      tunnel: w65 -> [w196]
      tunnel: [w194] -> w62
      tunnel: [w193] -> w60
      tunnel: w58 -> [w192]
      tunnel: [w192] -> w56
      tunnel: [w191] -> w49
      tunnel: w48 -> [_]
      tunnel: w124 -> [w228]
      tunnel: w123 -> [_]
      tunnel: w122 -> [w230]
      tunnel: [w230] -> w121
      tunnel: [w226] -> w120
      tunnel: w108 -> [w219]
      tunnel: [w228] -> w104
      tunnel: w102 -> [w227]
      tunnel: w98 -> [w225]
      tunnel: [w224] -> w94
      tunnel: w93 -> [w223]
      tunnel: [w222] -> w88
      tunnel: w82 -> [w221]
      tunnel: w80 -> [w217]
      tunnel: [w220] -> w75
      tunnel: w74 -> [w220]
      tunnel: w71 -> [w216]
      tunnel: [w213] -> w63
      tunnel: w62 -> [w213]
      tunnel: w60 -> [w212]
      tunnel: [w212] -> w59
      tunnel: w56 -> [w211]
      tunnel: [w211] -> w55
      tunnel: w49 -> [w210]
      tunnel: w121 -> [w247]
      tunnel: [w253] -> w105
      tunnel: w120 -> [w244]
      tunnel: [w249] -> w111
      tunnel: [w245] -> w79
      tunnel: w104 -> [w245]
      tunnel: [w244] -> w103
      tunnel: [w243] -> w95
      tunnel: w94 -> [w243]
      tunnel: [w242] -> w89
      tunnel: w88 -> [w242]
      tunnel: [w240] -> w76
      tunnel: w75 -> [w239]
      tunnel: w63 -> [w238]
      tunnel: [w238] -> w61
      tunnel: [w237] -> w51
      tunnel: w59 -> [w237]
      tunnel: w55 -> [w236]
      tunnel: [w236] -> w54
      frame #0 {
        n16 = call-poly <vilib>:"DAQmx Read.vi"("task/channels in"=w140, "error in"=w139) -> ("task out"=w135:refnum<k21>, "data"=w138:dbl, "error out"=w137:errorcluster)  [unwired: 11 in]
      }
      frame #1 {
        # "ÂoDC"
        n17 = Reciprocal(x=w155) -> (1/x=w154:dbl)
        n18 = Replace Array Subset(array=w176, new element=w152, index=0) -> (w157:dbl[])
        n19 = Bundle By Name("Y"=w157, "dt"=w154) -> (w164:waveform(dbl))  [unwired: 1 in]
        n20 = Add Array Elements(numeric array=w157) -> (sum=w175:dbl)
        n21 = Array Size(array=w157) -> (size(s)=w174:i32)
        n22 = call-poly <vilib>:"FFT Spectrum (Mag-Phase).vi"("averaging parameters"="averaging parameters", "time signal"=w164) -> ("magnitude"=w163:cluster{"f0":dbl, "df":dbl, "magnitude":dbl[]})  [unwired: 5 in, 4 out]
        "Waveform Graph" <- w163
        "magnitude" <- w163
        n23 = Divide(x=w175, y=w174) -> (x/y=w173:dbl)
        n24 = Multiply(x=w173, y=-1.0) -> (x*y=w171:dbl)
        n25 = Unbundle By Name(w163) -> ("magnitude"=w162:dbl[])
        n26 = Add(x=w171, y=w152) -> (x+y=w170:dbl)
        n27 = Replace Array Subset(array=w184, new element=w170, index=0) -> (w151:dbl[])
        n28 = Index Array(array=w162, index #1=4 ("index"), index #2=5 ("index")) -> (element #1=w159:dbl, element #2=w158:dbl)
        n29 = Greater Or Equal?(x=w159, y=w158) -> (x >= y?=w156:bool)
        "x >= y?" <- w156
        n30 = Split 1D Array(array=w151, index="平均數") -> (first subarray=w169:dbl[])  [unwired: 1 out]
        n31 = Add Array Elements(numeric array=w169) -> (sum=w168:dbl)
        n32 = case shown="False" w156 {
          frame False {
          }
          frame True {
          }
        }
        n33 = Divide(x=w168, y="平均數") -> (x/y=w148:dbl)
        n34 = Replace Array Subset(array=w151, new element=w148, index=0) -> (w150:dbl[])
      }
      frame #2 {
        # "積分誤差回朔"
        # "FIR"
        n35 = Multiply(x=w190, y=w188) -> (x*y=w205:dbl[])
        n36 = Add(x=w205, y=w204) -> (x+y=w203:dbl[])
        n37 = Add Array Elements(numeric array=w203) -> (sum=w189:dbl)
        n38 = Multiply(x=w189, y="Kp") -> (x*y=w201:dbl)
        n39 = Multiply(x=w201, y=1.0) -> (x*y=w186:dbl)
        n40 = call-poly <vilib>:"DAQmx Write.vi"("task/channels in"=w196, "data"=w186, "error in"=w195) -> ("task out"=w194:refnum<k21>, "error out"=w193:errorcluster)  [unwired: 10 in, 1 out]
      }
      frame #3 {
        # "ERR"
        n41 = Subtract(x=w221, y=w217) -> (x-y=w226:dbl)
        n42 = Multiply(x=w216, y="ÂoDC«á©ñ¤j") -> (x*y=w214:dbl)
        n43 = Build Array(w219, w216, w210) -> (w218:dbl[])
        n44 = Build Array(w217, w214) -> (w232:dbl[])
        n45 = call "積分器(SubVI).vi"("輸入累加ERR回朔"=w223, "I增益"="I增益", "samples (Hz)"=w225, "前一個ERR"=w227, "當下ERR"=w226) -> ("輸出累加ERR回朔"=w224:dbl, "積分修正量"=w222:dbl)  [unwired: 5 in]
        n46 = for {
          N: 1 -> [_]
          tunnel: [w235] -> w229 mode=indexing
          tunnel: w232 -> [w235]
          tunnel: [w234] -> w231 mode=indexing
          tunnel: w218 -> [w234]
        }
        "理想與FIR輸出" <- w229
        "模擬輸入x(t)" <- w231
      }
      frame #4 {
        n47 = Multiply(x="各頻率誤差低於多少亮燈", y=-1.0) -> (x*y=w250:dbl)
        n48 = In Range and Coerce(upper limit="各頻率誤差低於多少亮燈", x=w244, lower limit=w250) -> (In Range?=w246:bool)  [unwired: 1 out]
        "各頻率誤差已達標準" <- w246
        n49 = Rotate 1D Array(1:w247, 2:1 ("n")) -> (0:w253:dbl[])
        n50 = Rotate 1D Array(1:w239, 2:1 ("n")) -> (0:w240:dbl[])
        n51 = Not(x=w246) -> (.not. x?=w249:bool)
        "誤差" <- w244
        "當下誤差" <- w244
      }
    }
    n52 = call <vilib>:"High Resolution Relative Seconds.vi"() -> ("relative seconds"=w114:dbl)
    n53 = Subtract(x=w114, y=w112) -> (x-y=w119:dbl)
    n54 = Add(x=w119, y=w117) -> (x+y=w115:dbl)
    n55 = Divide(x=w115, y=w116) -> (x/y=→"while平均運行時間":dbl)
    n56 = case shown="True" w111 {
      tunnel: w113 -> [_ w132]
      frame False {
      }
      frame True {
        n57 = call <vilib>:"High Resolution Relative Seconds.vi"() -> ("relative seconds"=w134:dbl)
        n58 = Subtract(x=w134, y=w132) -> (x-y=→"收斂time":dbl)
      }
    }
    n59 = Unbundle By Name(w51) -> ("status"=w50:bool)
    n60 = Or(x=w50, y="stop") -> (x .or. y?=w53:bool)
  }
  n61 = call <vilib>:"DAQmx Stop Task.vi"("task/channels in"=w7, "error in"=w6) -> ("task out"=w8:refnum<k21>, "error out"=w9:errorcluster)  [unwired: 12 in]
  n62 = call <vilib>:"DAQmx Clear Task.vi"("task in"=w8, "error in"=w9) -> ("error out"=w12:errorcluster)  [unwired: 13 in]
  n63 = call <vilib>:"DAQmx Stop Task.vi"("task/channels in"=w5, "error in"=w12) -> ("task out"=w11:refnum<k21>, "error out"=w10:errorcluster)  [unwired: 12 in]
  n64 = call <vilib>:"DAQmx Clear Task.vi"("task in"=w11, "error in"=w10) -> ("error out"=w4:errorcluster)  [unwired: 13 in]
  n65 = call <vilib>:"Simple Error Handler.vi"("error in (no error)"=w4) -> ("message"=→"message":string)  [unwired: 4 in, 4 out]
